vi "PreserveNonWiredDataEnumToBools.vi"(11 "Preserve wired non-serialized data":T1) -> (2 "Preserve wired non-serialized data?":bool, 3 "Error on less-specific wired types?":bool)   [LabVIEW 2019, in "BlueSerialization.lvlib" / "BlueSerializer.lvclass"]
uses:
  BlueSerializer.lvclass
  PreserveNonWiredDataOption.ctl
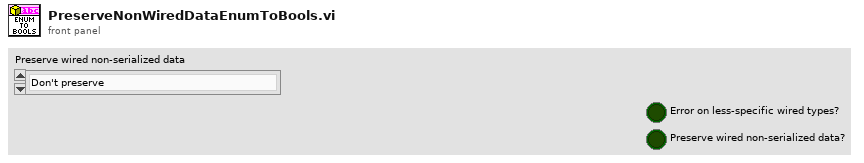
[diagram p1: front panel]
types:
  T1 = typedef "BlueSerialization.lvlib/BlueSerializer.lvclass/PreserveNonWiredDataOption.ctl" = enum16{"Don't preserve", "Preserve (error on less-specific wired types)", "Preserve (except on less-specific wired types)"}
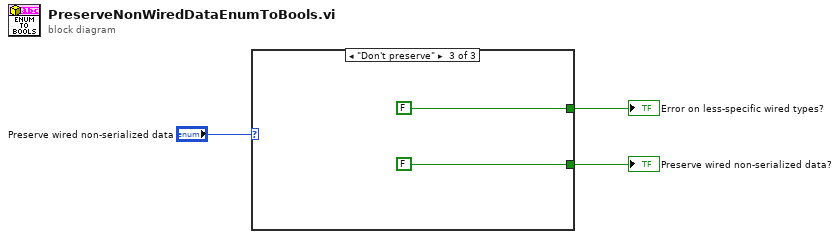
[diagram p0: block diagram]
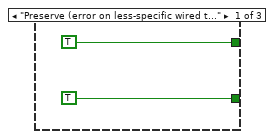
[diagram p2: hidden frame]
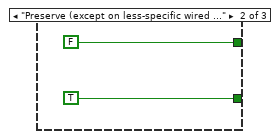
[diagram p3: hidden frame]
diagram:
  n1 = case shown="\"Don't preserve\"" "Preserve wired non-serialized data" {
    tunnel: [TRUE FALSE FALSE] -> w2
    tunnel: [TRUE TRUE FALSE] -> w1
    frame "Preserve (error on less-specific wired types)" {
    }
    frame "Preserve (except on less-specific wired types)" {
    }
    frame "Don't preserve" {
    }
  }
  "Preserve wired non-serialized data?" <- w1
  "Error on less-specific wired types?" <- w2
